vi "Stable_Rise&Fall.vi"(0 "Signal Input":bool, 1 "Rise Delay(sec)":dbl(knob)=0.5044674819294696 scale=0.0..1.0, 4 "Fall Delay(sec)":dbl(knob)=0.5044674819294696 scale=0.0..1.0) -> (7 "Stable":bool)   [LabVIEW 2016]
panel:
  out "Ready":bool
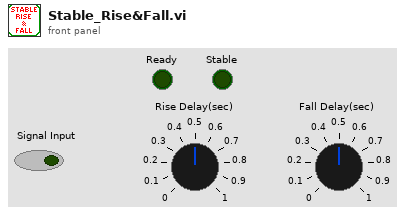
[diagram p1: front panel]
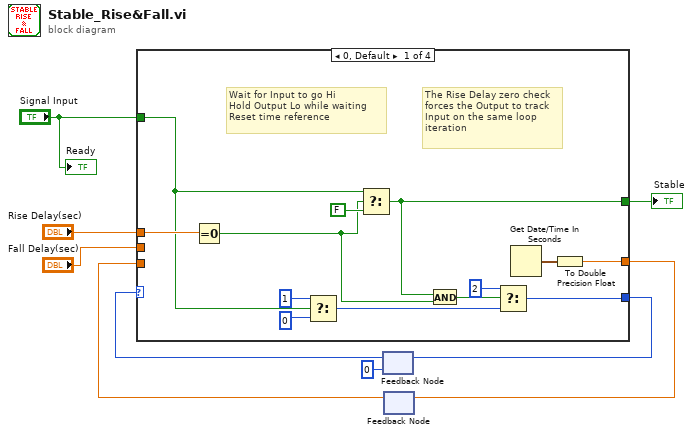
[diagram p0: block diagram]
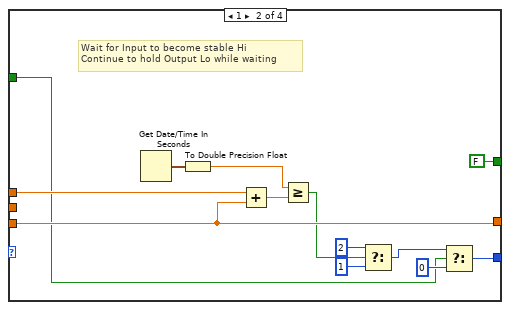
[diagram p2: hidden frame]
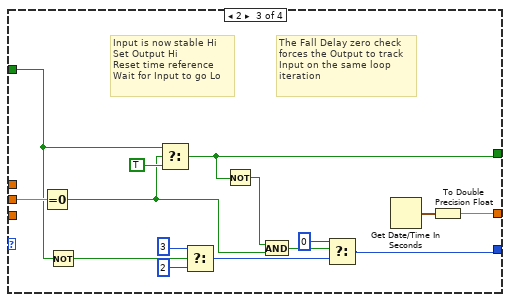
[diagram p3: hidden frame]
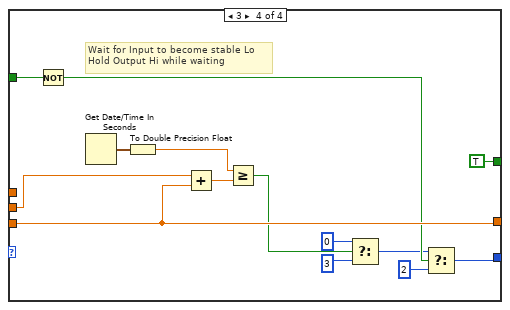
[diagram p4: hidden frame]
diagram:
  n1 = feedback #1(0 ("f")) -> (w9:i32)
  n2 = feedback #2() -> (w7:dbl)  [unwired: 1 in]
  n3 = case shown="0, Default" w9 {
    tunnel: [w13 w23 w40 w55] -> w3
    tunnel: "Signal Input" -> [w17 w26 w43 w62]
    tunnel: [w12 FALSE w37 TRUE] -> w4
    tunnel: [w19 w33 w49 w58] -> w8
    tunnel: w7 -> [_ w33 _ w58]
    tunnel: "Rise Delay(sec)" -> [w18 w34 _ _]
    tunnel: "Fall Delay(sec)" -> [_ _ w46 w57]
    frame 0, Default {
      # "The Rise Delay zero check\nforces the Output to track\nInput on the same loop\niteration"
      # "Wait for Input to go Hi\nHold Output Lo while waiting\nReset time reference"
      n4 = Equal To 0?(x=w18) -> (x = 0?=w11:bool)
      n5 = Select(t=1, s=w17, f=0) -> (s? t:f=w15:i32)
      n6 = Select(t=w17, s=w11, f=FALSE) -> (s? t:f=w12:bool)
      n7 = And(x=w12, y=w11) -> (x .and. y?=w10:bool)
      n8 = Select(t=2, s=w10, f=w15) -> (s? t:f=w13:i32)
      n9 = Get Date/Time In Seconds() -> (seconds since 1Jan1904=w20:timestamp)
      n10 = To Double Precision Float(number=w20) -> (double precision float=w19:dbl)
    }
    frame 1 {
      # "Wait for Input to become stable Hi\nContinue to hold Output Lo while waiting"
      n11 = Get Date/Time In Seconds() -> (seconds since 1Jan1904=w35:timestamp)
      n12 = To Double Precision Float(number=w35) -> (double precision float=w31:dbl)
      n13 = Add(x=w34, y=w33) -> (x+y=w32:dbl)
      n14 = Greater Or Equal?(x=w31, y=w32) -> (x >= y?=w29:bool)
      n15 = Select(t=2, s=w29, f=1) -> (s? t:f=w24:i32)
      n16 = Select(t=w24, s=w26, f=0) -> (s? t:f=w23:i32)
    }
    frame 2 {
      # "The Fall Delay zero check\nforces the Output to track\nInput on the same loop\niteration"
      # "Input is now stable Hi\nSet Output Hi\nReset time reference\nWait for Input to go Lo"
      n17 = Equal To 0?(x=w46) -> (x = 0?=w39:bool)
      n18 = Not(x=w43) -> (.not. x?=w44:bool)
      n19 = Select(t=w43, s=w39, f=TRUE) -> (s? t:f=w37:bool)
      n20 = Select(t=3, s=w44, f=2) -> (s? t:f=w42:i32)
      n21 = Not(x=w37) -> (.not. x?=w36:bool)
      n22 = And(x=w36, y=w39) -> (x .and. y?=w38:bool)
      n23 = Select(t=0, s=w38, f=w42) -> (s? t:f=w40:i32)
      n24 = Get Date/Time In Seconds() -> (seconds since 1Jan1904=w50:timestamp)
      n25 = To Double Precision Float(number=w50) -> (double precision float=w49:dbl)
    }
    frame 3 {
      # "Wait for Input to become stable Lo\nHold Output Hi while waiting"
      n26 = Not(x=w62) -> (.not. x?=w54:bool)
      n27 = Get Date/Time In Seconds() -> (seconds since 1Jan1904=w61:timestamp)
      n28 = To Double Precision Float(number=w61) -> (double precision float=w59:dbl)
      n29 = Add(x=w57, y=w58) -> (x+y=w60:dbl)
      n30 = Greater Or Equal?(x=w59, y=w60) -> (x >= y?=w51:bool)
      n31 = Select(t=0, s=w51, f=3) -> (s? t:f=w53:i32)
      n32 = Select(t=w53, s=w54, f=2) -> (s? t:f=w55:i32)
    }
  }
  "Stable" <- w4
  n33 = feedback-in #1(w3) -> ()
  n34 = feedback-in #2(w8) -> ()
  "Ready" <- "Signal Input"
